vi "Example 3.vi"() -> ()   [LabVIEW 2018]
uses:
  <vilib>/addons/VeriStand Custom Device Scripting APIs/FPGA Addon/Scripting API.lvlibp/APIs/Scripting API/TypeDefs/Output Scalar Data.ctl
  <vilib>/addons/VeriStand Custom Device Scripting APIs/FPGA Addon/Scripting API.lvlibp/Addon/Addon Shared/Types/Data Type.ctl
  <vilib>/addons/VeriStand Custom Device Scripting APIs/FPGA Addon/Scripting API.lvlibp/APIs/Scripting API/Public/Bitfile Resources/Import Bitfile Scalars (Instances)/Import Scalars - all.vi
  <vilib>/addons/VeriStand Custom Device Scripting APIs/FPGA Addon/Scripting API.lvlibp
  <vilib>/addons/VeriStand Custom Device Scripting APIs/FPGA Addon/Scripting API.lvlibp/Addon/Addon Shared/FPGA Addon Shared.lvlib
panel:
  out "imported bitfile scalars out":T1[](array[typedef])
  out "error out":errorcluster
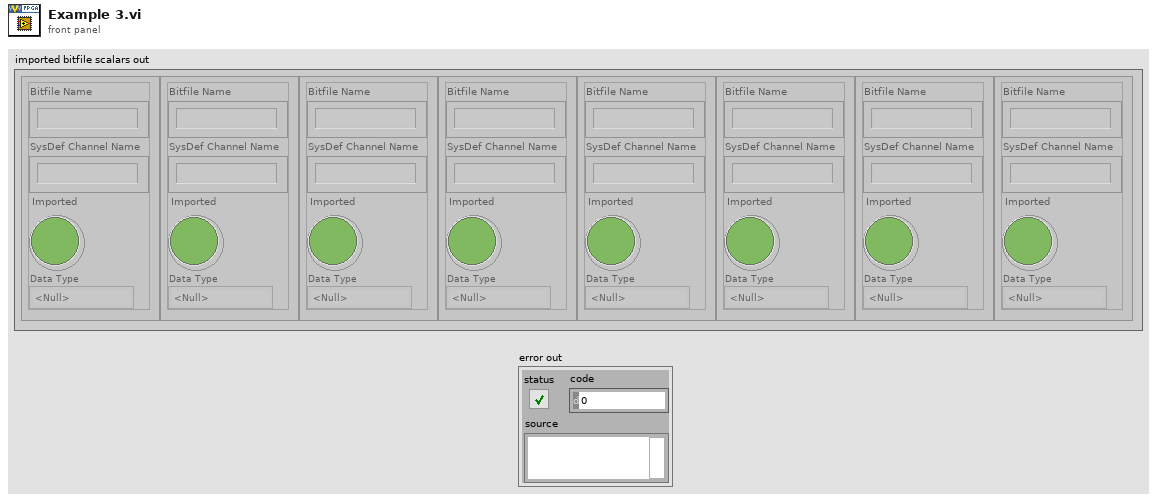
[diagram p1: front panel]
types:
  T1 = typedef "Scripting API.lvlibp/Output Scalar Data.ctl" = cluster{"Bitfile Name":string, "SysDef Channel Name":string, "Imported":bool, "Data Type":T2}
  T2 = typedef "Scripting API.lvlibp/FPGA Addon Shared.lvlib/Data Type.ctl" = enum8{"<Null>", "I8", "I16", "I32", "I64", "U8", "U16", "U32", "U64", "SGL", "Boolean", "Analog PWM In Settings", "Analog PWM In", "Digital PWM In Settings", "Digital PWM In", "Digital PWM Out", "Sine Out", "FXP+/-24.5", "FXP+/-16.5", "FXP+/-32.8", "FXP+/-64.32", "FXP+/-16.7", "FXP+/-20.5", "FXP+/-27.5", "FXP+/-32.16", "FXP+16.3", "FXP+18.3", "Digital Static In", "Digital Static Out", "Digital Static In Settings", "Digital WSS Out", "Quad Encoder Settings", "Quad Encoder In", "Group"}
  T3 = typedef "Scripting API.lvlibp/Custom Device API.lvlib/Custom Device Item Ref.ctl" = u64
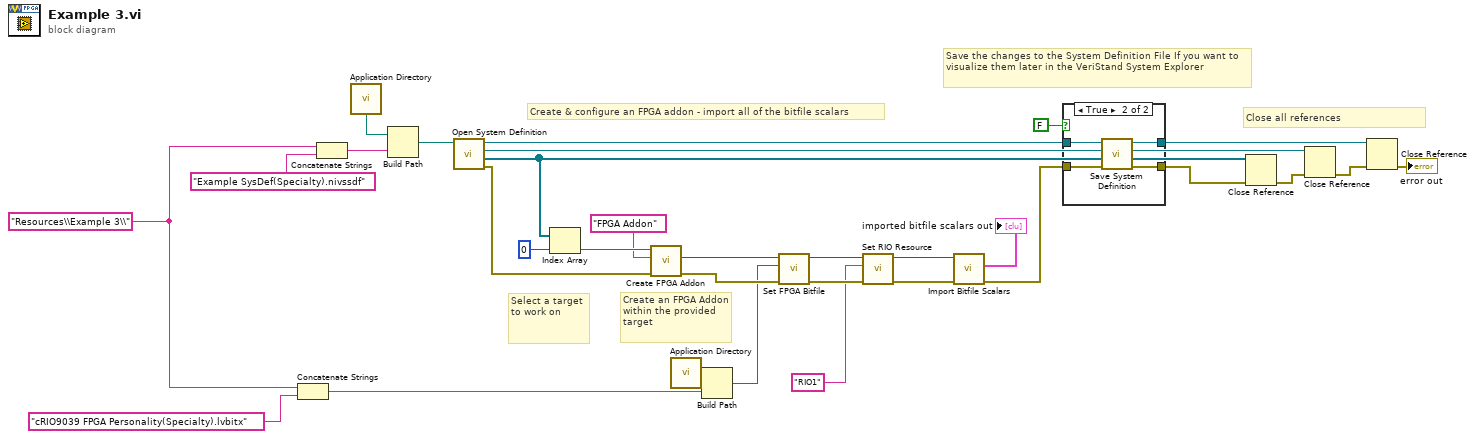
[diagram p0: block diagram]
diagram:
  w14 = "Resources\\Example 3\\" ("name or relative path")
  # "Create & configure an FPGA addon - import all of the bitfile scalars"
  # "Save the changes to the System Definition File If you want to visualize them later in the VeriStand System Explorer"
  # "Close all references"
  # "Create an FPGA Addon within the provided target"
  # "Select a target to work on"
  n1 = Concatenate Strings(w14, "cRIO9039 FPGA Personality(Specialty).lvbitx" ("name or relative path")) -> (w12:string)
  n2 = Concatenate Strings(w14, "Example SysDef(Specialty).nivssdf" ("name or relative path")) -> (w15:string)
  n3 = call <vilib>:"Application Directory.vi"() -> ("Application Directory"=w26:path)
  n4 = Build Path(base path=w26, name or relative path=w15) -> (appended path=w25:path)
  n5 = call "Open System Definition.vi"("System Definition File"=w25) -> ("error out"=w17:errorcluster, "targets refnums"=w29:refnum<k24>[], "root refnum"=w30:refnum<k24>, "system definition refnum"=w23:refnum<k24>)  [unwired: 7 in]
  n6 = Index Array(array=w29, index=0) -> (element=w19:refnum<k24>)
  n7 = call <vilib>:"Create FPGA Addon.vi"("error in"=w17, "FPGA addon name"="FPGA Addon" ("fpga addon name"), "target in"=w19) -> ("error out"=w10:errorcluster, "FPGA addon refnum"=w9:T3)  [unwired: 6 in, 1 out]
  n8 = call <vilib>:"Application Directory.vi"() -> ("Application Directory"=w20:path)
  n9 = Build Path(base path=w20, name or relative path=w12) -> (appended path=w8:path)
  n10 = call <vilib>:"Set FPGA Bitfile.vi"("error in"=w10, "FPGA bitfile path"=w8, "FPGA addon refnum in"=w9) -> ("error out"=w7:errorcluster, "FPGA addon refnum out"=w6:T3)  [unwired: 7 in]
  n11 = call <vilib>:"Set RIO Resource.vi"("error in"=w7, "RIO resource in"="RIO1", "FPGA addon refnum in"=w6) -> ("error out"=w4:errorcluster, "FPGA addon refnum out"=w3:T3)  [unwired: 7 in]
  n12 = call-poly <vilib>:"Import Bitfile Scalars.vi"("error in"=w4, "FPGA addon refnum in"=w3) -> ("error out"=w2:errorcluster, "imported bitfile scalars out"=→"imported bitfile scalars out":T1[])  [unwired: 7 in, 1 out]
  n13 = case shown="True" FALSE {
    tunnel: w23 -> [w33 w37]
    tunnel: [w33 w36] -> w22
    tunnel: [w32 w35] -> w21
    tunnel: w2 -> [w32 w34]
    frame False {
    }
    frame True {
      n14 = call "Save System Definition.vi"("error in (no error)"=w34, ".NET Refnum in"=w37) -> ("error out"=w35:errorcluster, ".NET Refnum out"=w36:refnum<k24>)  [unwired: 8 in]
    }
  }
  n15 = Close Reference(reference=w29, error in (no error)=w21) -> (error out=w28:errorcluster)
  n16 = Close Reference(reference=w30, error in (no error)=w28) -> (error out=w27:errorcluster)
  n17 = Close Reference(reference=w22, error in (no error)=w27) -> (error out=→"error out":errorcluster)
